vi "PopulateSheduledStatusOfDosages.vi"(8 "error in":errorcluster, 9 "StartTimeOfDrugController":timestamp, 10 "Array":timestamp[](array[timestamp]), 11 "Array 2":refnum<vi>[](array[refnum])) -> (0 "error out":errorcluster)   [LabVIEW 2019]
uses:
  DrugDosageTimeStampReference.ctl
  <vilib>/regexp/Match Regular Expression.xnode
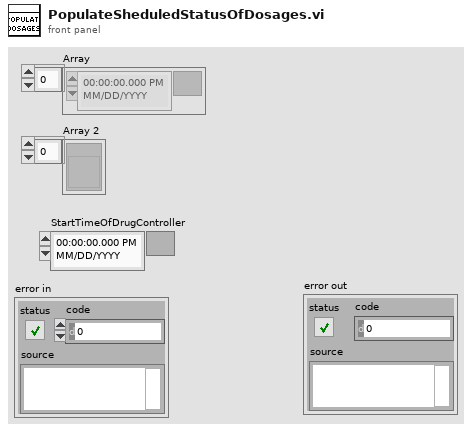
[diagram p1: front panel]
types:
  T1 = typedef "DrugDosageTimeStampReference.ctl" = cluster{"TimeStampControlReference":refnum<vi>, "DosageTime":timestamp}
  T2 = enum8{"Enabled", "Disabled", "Disabled and Grayed Out"}
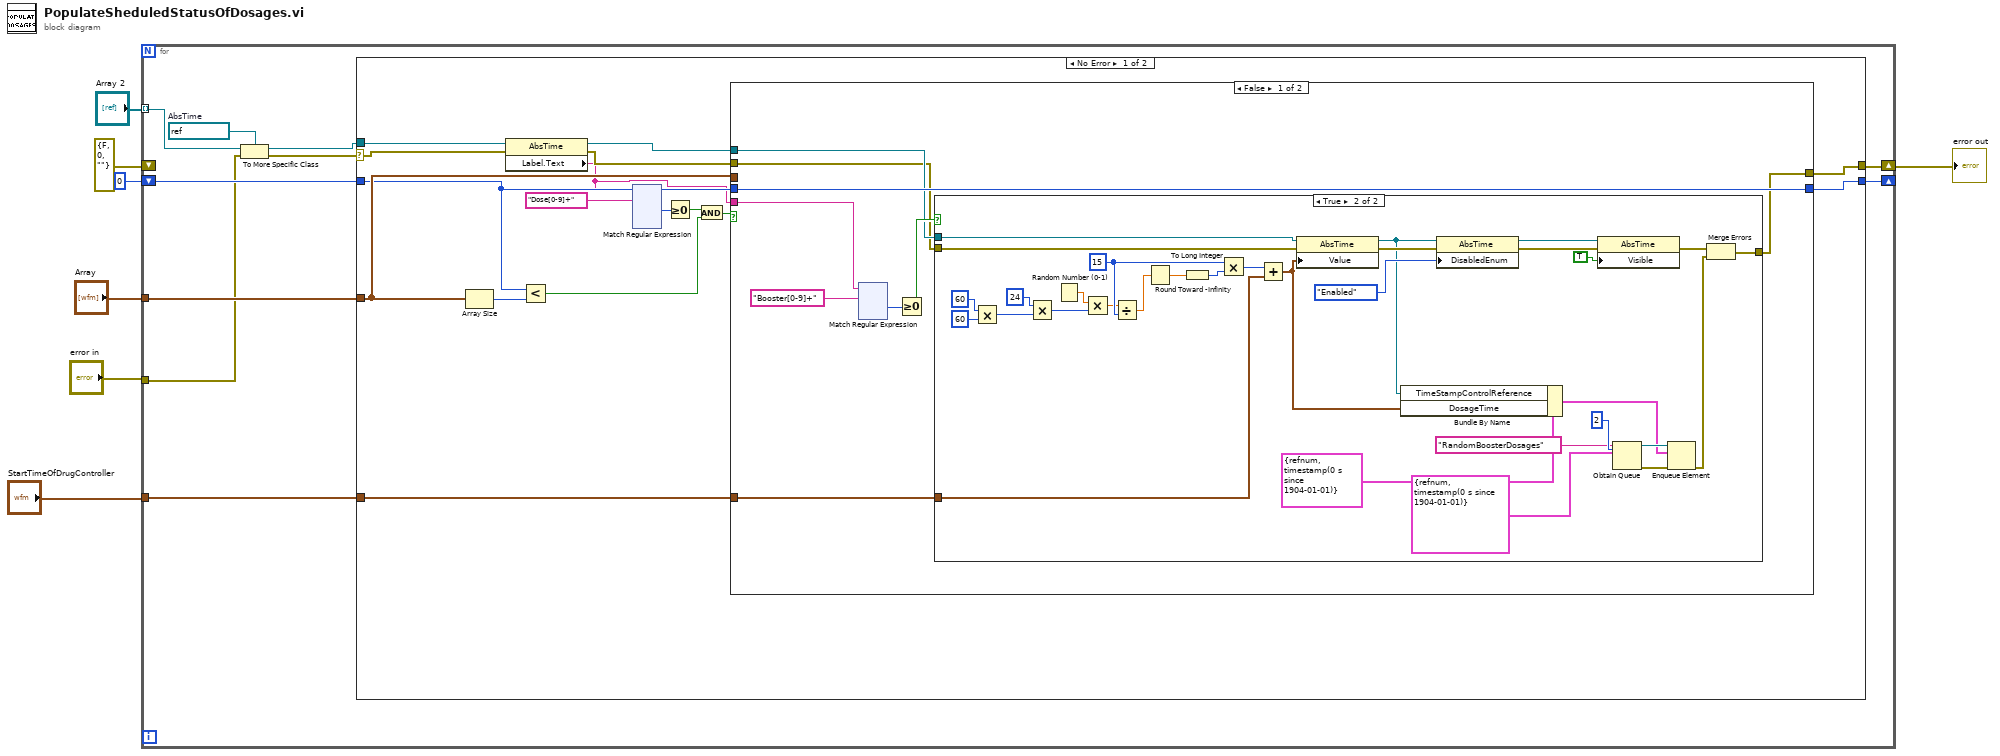
[diagram p0: block diagram]
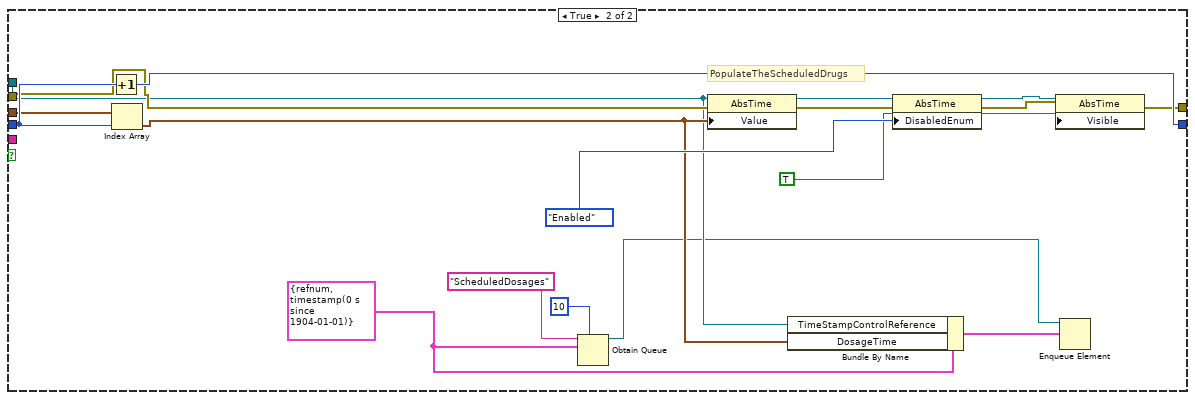
[diagram p3: hidden frame]
diagram:
  n1 = for {
    tunnel: "Array 2" -> [w13] mode=indexing
    tunnel: "Array" -> [w17]
    shift-right: [w15] -> _
    shift-left: 0 -> [w16]
    tunnel: "error in" -> [w10]
    shift-right: [w9] -> w2
    shift-left: errorcluster {"status"=FALSE, "code"=0, "source"=""} ("error out") -> [_]
    tunnel: "StartTimeOfDrugController" -> [w8]
    w14 = refnum<vi> refnum  # AbsTime
    n2 = To More Specific Class(target class=w14, reference=w13, error in=w10) -> (specific class reference=w12:refnum<vi>, error out=w11:errorcluster)
    n3 = case shown="No Error" w11 {
      selector: w11 -> [w21 _]
      tunnel: w17 -> [w27 _]
      tunnel: w16 -> [w26 w324]
      tunnel: [w32 w324] -> w15
      tunnel: w12 -> [w31 _]
      tunnel: [w20 _] -> w9
      tunnel: w8 -> [w18 _]
      frame No Error {
        n4 = Array Size(array=w27) -> (size(s)=w25:i32)
        n5 = property class="AbsTime"(reference=w31, error in=w21) -> (reference out=w33:refnum<vi>, error out=w22:errorcluster, "Label.Text"=w19:string)
        n6 = Less?(x=w26, y=w25) -> (x < y?=w24:bool)
        n7 = xnode "Match Regular Expression"("input string"=w19, "regular expression"="Dose[0-9]+") -> ("offset past match"=w29:i32)  [unwired: 4 in, 5 out]
        n8 = Greater Or Equal To 0?(x=w29) -> (x >= 0?=w28:bool)
        n9 = And(x=w28, y=w24) -> (x .and. y?=w23:bool)
        n10 = case shown="False" w23 {
          tunnel: w33 -> [w153 w308]
          tunnel: w27 -> [_ w318]
          tunnel: w26 -> [w158 w319]
          tunnel: [w158 w317] -> w32
          tunnel: w22 -> [w151 w316]
          tunnel: [w150 w313] -> w20
          tunnel: w19 -> [w156 _]
          tunnel: w18 -> [w152 _]
          frame False {
            n11 = xnode "Match Regular Expression"("input string"=w156, "regular expression"="Booster[0-9]+") -> ("offset past match"=w155:i32)  [unwired: 4 in, 4 out]
            n12 = Greater Or Equal To 0?(x=w155) -> (x >= 0?=w154:bool)
            n13 = case shown="True" w154 {
              tunnel: w153 -> [_ w182]
              tunnel: w152 -> [_ w177]
              tunnel: w151 -> [w159 w165]
              tunnel: [w159 w161] -> w150
              frame False {
              }
              frame True {
                w185 = u32 15 ("y")
                n14 = Multiply(x=60, y=60) -> (x*y=w175:i32)
                n15 = Multiply(x=24, y=w175) -> (x*y=w174:i32)
                n16 = Random Number (0-1)() -> (number: 0 to 1=w181:dbl)
                n17 = Multiply(x=w181, y=w174) -> (x*y=w178:dbl)
                n18 = Divide(x=w178, y=w185) -> (x/y=w183:dbl)
                n19 = Round Toward -Infinity(1:w183) -> (0:w184:dbl)
                n20 = To Long Integer(number=w184) -> (32bit integer=w186:i32)
                n21 = Multiply(x=w185, y=w186) -> (x*y=w187:u32)
                n22 = Add(x=w187, y=w177) -> (x+y=w168:timestamp)
                n23 = property class="AbsTime"(reference=w182, error in=w165, "Value"=w168) -> (reference out=w169:refnum<vi>, error out=w188:errorcluster)
                n24 = Bundle By Name(cluster=T1 {"TimeStampControlReference"=refnum, "DosageTime"=timestamp(0 s since 1904-01-01)}, "TimeStampControlReference"=w169, "DosageTime"=w168) -> (w160:T1)
                n25 = property class="AbsTime"(reference=w169, error in=w188, "DisabledEnum"=T2."Enabled" ("Disabled")) -> (reference out=w191:refnum<vi>, error out=w166:errorcluster)
                n26 = property class="AbsTime"(reference=w191, error in=w166, "Visible"=TRUE) -> (error out=w164:errorcluster)  [unwired: 1 out]
                n27 = Obtain Queue(max queue size (-1, unlimited)=2, name (unnamed)="RandomBoosterDosages", element data type=T1 {"TimeStampControlReference"=refnum, "DosageTime"=timestamp(0 s since 1904-01-01)}) -> (queue out=w167:refnum<queue>, error out=w163:errorcluster)  [unwired: 2 in, 1 out]
                n28 = Enqueue Element(queue=w167, element=w160, error in (no error)=w163) -> (error out=w162:errorcluster)  [unwired: 1 in, 2 out]
                n29 = Merge Errors(w164, w162) -> (w161:errorcluster)
              }
            }
          }
          frame True {
            w310 = T1 {"TimeStampControlReference"=refnum, "DosageTime"=timestamp(0 s since 1904-01-01)}
            # "PopulateTheScheduledDrugs"
            n30 = Increment(x=w319) -> (x+1=w317:i32)
            n31 = Index Array(array=w318, index=w319) -> (element=w309:timestamp)
            n32 = Obtain Queue(max queue size (-1, unlimited)=10, name (unnamed)="ScheduledDosages", element data type=w310) -> (queue out=w306:refnum<queue>)  [unwired: 2 in, 2 out]
            n33 = property class="AbsTime"(reference=w308, error in=w316, "Value"=w309) -> (reference out=w322:refnum<vi>, error out=w315:errorcluster)
            n34 = Bundle By Name(cluster=w310, "TimeStampControlReference"=w308, "DosageTime"=w309) -> (w307:T1)
            n35 = property class="AbsTime"(reference=w322, error in=w315, "DisabledEnum"=T2."Enabled" ("Disabled")) -> (reference out=w321:refnum<vi>, error out=w314:errorcluster)
            n36 = property class="AbsTime"(reference=w321, error in=w314, "Visible"=TRUE) -> (error out=w313:errorcluster)  [unwired: 1 out]
            n37 = Enqueue Element(queue=w306, element=w307) -> ()  [unwired: 2 in, 3 out]
          }
        }
      }
      frame Error {
      }
    }
  }
  "error out" <- w2
